vi "XY图调用节点导出图像.vi"() -> ()   [LabVIEW 2014]
panel:
  in  "导出图像":bool
  out "XY图":cluster{dbl[], dbl[]}(graph)
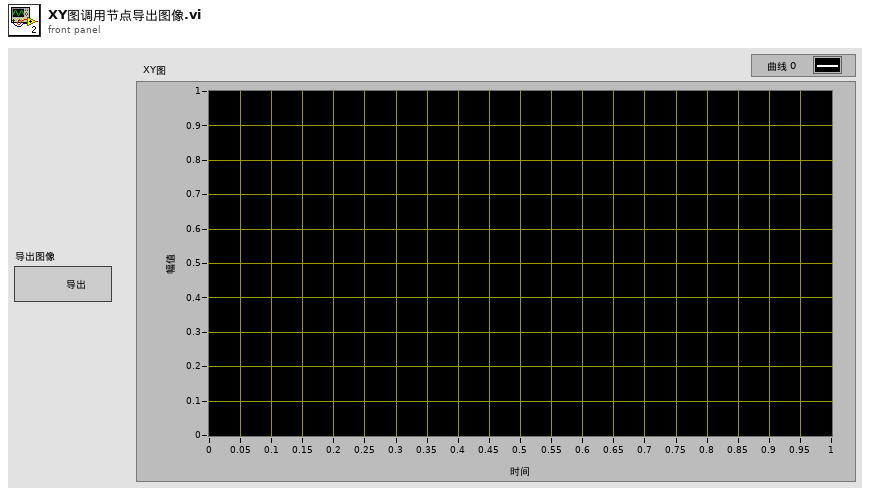
[diagram p1: front panel]
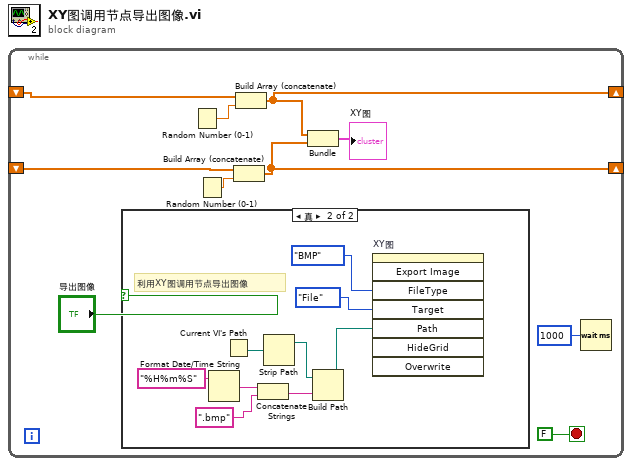
[diagram p0: block diagram]
diagram:
  n1 = while {
    shift-right: [w7] -> _
    shift-left: _ -> [w5]
    shift-right: [w3] -> _
    shift-left: _ -> [w2]
    stop <- FALSE stop-if-true
    n2 = case shown="真" "导出图像" {
      frame False {
      }
      frame True {
        # "利用XY图调用节点导出图像"
        n3 = Format Date/Time String(time format string (%c)="%H%m%S" ("时间格式字符串(%c)")) -> (date/time string=w13:string)  [unwired: 2 in]
        n4 = Current VI's Path() -> (path=w16:path)
        n5 = Concatenate Strings(w13, ".bmp" ("字符串")) -> (w14:string)
        n6 = Strip Path(path=w16) -> (stripped path=w15:path)  [unwired: 1 out]
        n7 = Build Path(base path=w15, name or relative path=w14) -> (appended path=w12:path)
        n8 = invoke on="XY图" class="XYGraph (严格)" method="Export Image"("FileType"=enum32{"BMP", "EPS", "EMF", "PICT"}."BMP" ("文件类型"), "Target"=enum32{"File", "Clipboard"}."File" ("目标"), "Path"=w12) -> ()  [unwired: 5 in, 8 out]
      }
    }
    n9 = Random Number (0-1)() -> (number: 0 to 1=w6:dbl)
    n10 = Random Number (0-1)() -> (number: 0 to 1=w4:dbl)
    n11 = Build Array (concatenate)(w2, w4) -> (w3:dbl[])
    n12 = Build Array (concatenate)(w5, w6) -> (w7:dbl[])
    n13 = Bundle(w7, w3) -> (→"XY图":cluster{dbl[], dbl[]})  [unwired: 1 in]
    n14 = Wait (ms)(milliseconds to wait=u32 1000 ("等待时间（毫秒）")) -> ()  [unwired: 1 out]
  }
